vi "Unpack Gamepad.vi"(11 "JoystickDevRef":T1) -> (0 "Button Array":bool[](array[boolean]), 2 "Button Cluster":T4, 3 "Axes":T5, 5 "POV":T3)   [LabVIEW 2014]
uses:
  <vilib>/Rock Robotics/WPI/Joystick/WPI_JoystickDevRef.ctl
  <vilib>/Rock Robotics/WPI/Joystick/WPI_JoystickDeviceEnum.ctl
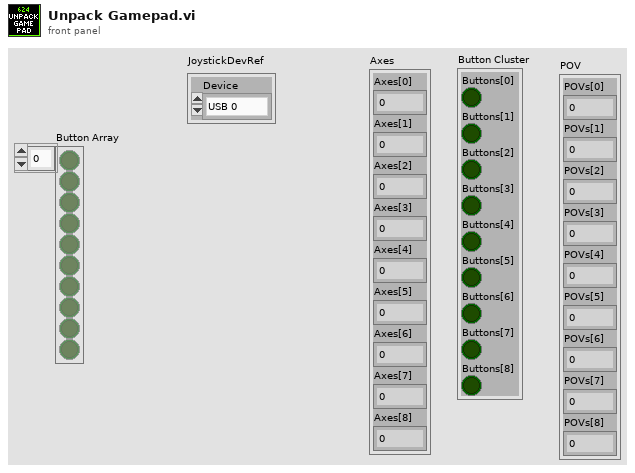
[diagram p1: front panel]
types:
  T1 = typedef "WPI_JoystickDevRef.ctl" = cluster{"Device":T2}
  T2 = typedef "WPI_JoystickDeviceEnum.ctl" = enum16{"USB 0", "USB 1", "USB 2", "USB 3", "USB 4", "USB 5"}
  T3 = cluster{"POVs[0]":i16, "POVs[1]":i16, "POVs[2]":i16, "POVs[3]":i16, "POVs[4]":i16, "POVs[5]":i16, "POVs[6]":i16, "POVs[7]":i16, "POVs[8]":i16}
  T4 = cluster{"Buttons[0]":bool, "Buttons[1]":bool, "Buttons[2]":bool, "Buttons[3]":bool, "Buttons[4]":bool, "Buttons[5]":bool, "Buttons[6]":bool, "Buttons[7]":bool, "Buttons[8]":bool}
  T5 = cluster{"Axes[0]":dbl, "Axes[1]":dbl, "Axes[2]":dbl, "Axes[3]":dbl, "Axes[4]":dbl, "Axes[5]":dbl, "Axes[6]":dbl, "Axes[7]":dbl, "Axes[8]":dbl}
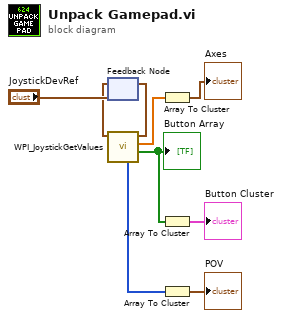
[diagram p0: block diagram]
diagram:
  n1 = feedback #1("JoystickDevRef") -> (w3:T1)
  n2 = call <vilib>:"WPI_JoystickGetValues.vi"("JoystickDevRef"=w3) -> ("Buttons"=w2:bool[], "Axes"=w9:dbl[], "JoystickDevRef"=w4:T1, "POVs"=w7:i16[])  [unwired: 6 in, 1 out]
  "Button Array" <- w2
  n3 = feedback-in #1(w4) -> ()
  n4 = Array To Cluster(array=w9) -> (cluster=→"Axes":T5)
  n5 = Array To Cluster(array=w2) -> (cluster=→"Button Cluster":T4)
  n6 = Array To Cluster(array=w7) -> (cluster=→"POV":T3)
